vi "MoveMotors2.vi"(8 "error in (no error)":errorcluster, 9 "Target":dbl[](array[numeric]), 10 "N Ax":dbl, 11 "CU ID":i32) -> (0 "error out":errorcluster)   [LabVIEW 2021]
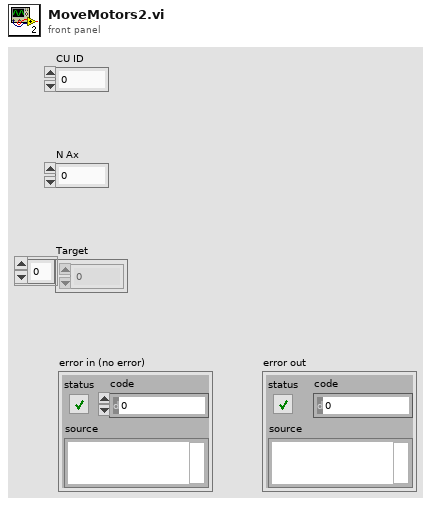
[diagram p1: front panel]
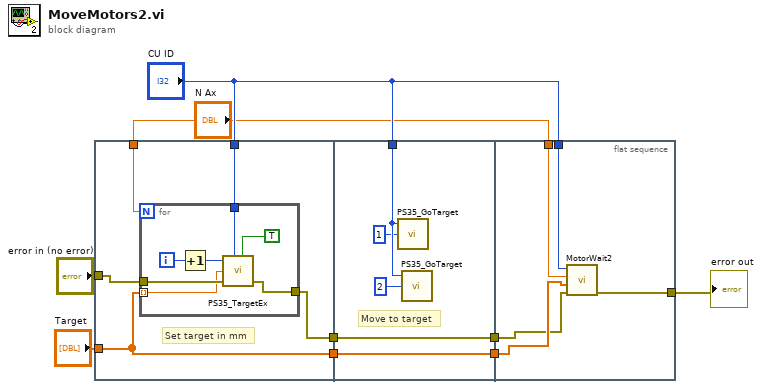
[diagram p0: block diagram]
diagram:
  n1 = flat-sequence {
    tunnel: "error in (no error)" -> [w14]
    tunnel: "CU ID" -> [w12]
    tunnel: "N Ax" -> [w13]
    tunnel: [w11] -> w9
    tunnel: "Target" -> [w10]
    tunnel: [w10] -> w4
    tunnel: "CU ID" -> [w26]
    tunnel: [w23] -> w8
    tunnel: w9 -> [w23]
    tunnel: [w22] -> w5
    tunnel: w4 -> [w22]
    tunnel: w8 -> [w28]
    tunnel: "N Ax" -> [w30]
    tunnel: "CU ID" -> [w31]
    tunnel: w5 -> [w29]
    tunnel: [w27] -> w1
    frame #0 {
      # "Set target in mm"
      n2 = for {
        N: w13 -> [_]
        tunnel: [w18] -> w11
        tunnel: w14 -> [w17]
        tunnel: w12 -> [w16]
        tunnel: w10 -> [w15] mode=indexing
        i -> [w21]
        n3 = Increment(x=w21) -> (x+1=w19:i32)
        n4 = call "PS35_TargetEx.vi"("Axis number"=w19, "Control unit ID"=w16, "dValue-In"=w15, "error in (no error)"=w17, "function"=TRUE) -> ("error out"=w18:errorcluster)  [unwired: 3 in, 1 out]
      }
    }
    frame #1 {
      # "Move to target"
      n5 = call "PS35_GoTarget.vi"("Axis number"=1, "Control unit ID"=w26) -> ()  [unwired: 2 in, 1 out]
      n6 = call "PS35_GoTarget.vi"("Axis number"=2, "Control unit ID"=w26) -> ()  [unwired: 2 in, 1 out]
    }
    frame #2 {
      n7 = call "MotorWait2.vi"("error in (no error)"=w28, "Intended Position"=w29, "N Ax"=w30, "CU ID"=w31) -> ("error out"=w27:errorcluster)  [unwired: 7 in]
    }
  }
  "error out" <- w1
